vi "Session open.vi"(8 "error in":errorcluster, 11 "measurement configuration":T1={"INTERFACE NAME CAN"="", "IO Mode CAN"=enum."CAN", "FD ISO Mode CAN"=enum."ISO", "Termination CAN"=FALSE, "Baudrate CAN"=0, "FD Baudrate CAN"=0, "INTERFACE NAME LIN"="", "Termination LIN"=FALSE, "CAN interface"="", "LIN interface"="", "Network"="", "DLC INDICATOR"=0, "PAYLOAD INDICATOR"=[0, 0, 0, 0, 0, 0, 0, 0, 0, 0, 0, 0, 0, 0, 0, 0, 0, 0, 0, 0, 0, 0, 0, 0, 0, 0, 0, 0, 0, 0, 0, 0, 0, 0, 0, 0, 0, 0, 0, 0, 0, 0, 0, 0, 0, 0, 0, 0, 0, 0, 0, 0, 0, 0, 0, 0, 0, 0, 0, 0, 0, 0, 0, 0], "IDENTIFIER INDICATOR"=0, "Baudrate LIN"=0} {"Baudrate LIN" format="%x"; "IDENTIFIER INDICATOR" format="%x"; "PAYLOAD INDICATOR" format="%x"; "FD Baudrate CAN" format="%x"; "Baudrate CAN" format="%x"}) -> (0 "error out":errorcluster, 3 "session out":refnum<k21>)   [LabVIEW 2025, in "CAN-LIN Frame Generator.lvclass"]
uses:
  CAN-LIN Frame Generator.lvclass
  Measurement Configuration.ctl
  CAN-LIN Frame Generator UI/Toggle.ctl
  <vilib>/xnet/xnet.llb/XNET Create Session (Frame Output Stream).vi
  CAN-LIN Frame Generator.lvclass/CAN-LIN Frame Generator.ctl
  <resource>/objmgr/xnet.rc
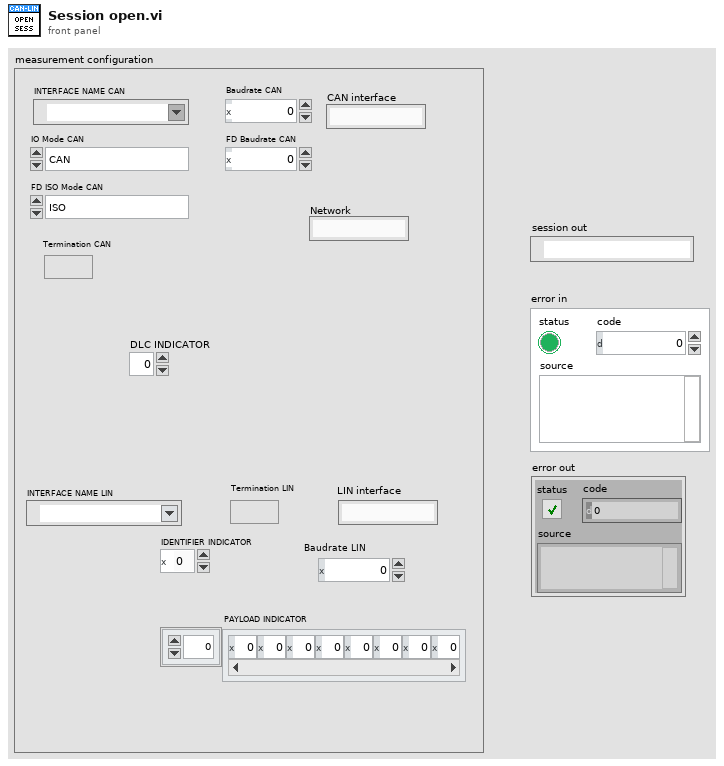
[diagram p1: front panel]
types:
  T1 = typedef "CAN-LIN Frame Generator.lvclass/Measurement Configuration.ctl" = cluster{"INTERFACE NAME CAN":refnum<k21>, "IO Mode CAN":enum32{"CAN", "CAN FD", "CAN FD + BRS"}, "FD ISO Mode CAN":enum32{"ISO", "Legacy ISO", "Non-ISO"}, "Termination CAN":T2, "Baudrate CAN":u32, "FD Baudrate CAN":u32, "INTERFACE NAME LIN":refnum<k21>, "Termination LIN":T2, "CAN interface":string, "LIN interface":string, "Network":string, "DLC INDICATOR":u32, "PAYLOAD INDICATOR":u32[], "IDENTIFIER INDICATOR":u32, "Baudrate LIN":u32}
  T2 = typedef "Toggle.ctl" = bool
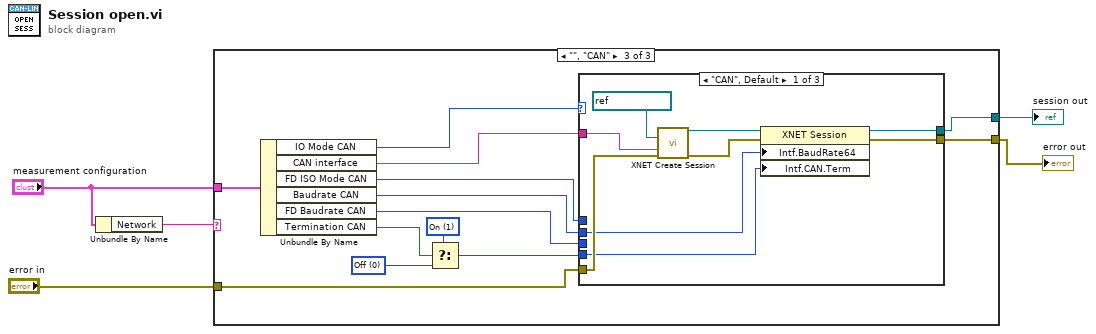
[diagram p0: block diagram]
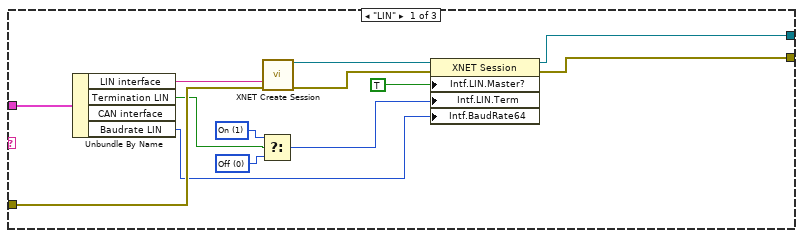
[diagram p2: hidden frame]
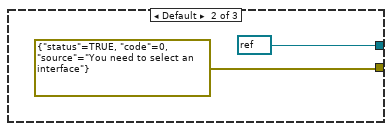
[diagram p3: hidden frame]
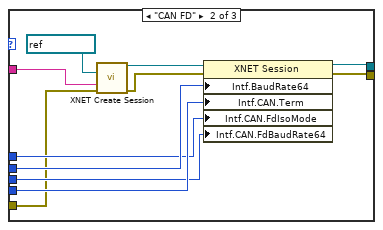
[diagram p4: hidden frame]
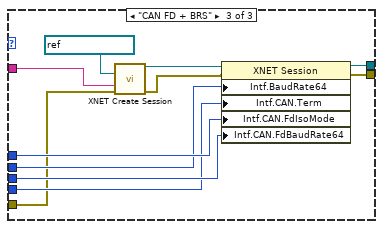
[diagram p5: hidden frame]
diagram:
  n1 = Unbundle By Name("measurement configuration") -> ("Network"=w1:string)
  n2 = case shown="\"\", \"CAN\"" w1 {
    tunnel: "error in" -> [w16 _ w30]
    tunnel: [w8 refnum<k21> refnum ("session out") w23] -> w4
    tunnel: [w7 errorcluster {"status"=TRUE, "code"=0, "source"="You need to select an interface"} ("error out") w22] -> w3
    tunnel: "measurement configuration" -> [w18 _ w21]
    frame "LIN" {
      w11 = u32 0 items=["Off", "On"] ("Interface:LIN:Termination")
      w12 = u32 1 items=["Off", "On"] ("Interface:LIN:Termination")
      n3 = Unbundle By Name(w18) -> ("LIN interface"=w17:string, "Termination LIN"=w13:T2, "Baudrate LIN"=w6:u32)  [unwired: 1 out]
      n4 = Select(t=w12, s=w13, f=w11) -> (s? t:f=w10:u32)
      n5 = call-poly <vilib>:"XNET Create Session.vi"("interface"=w17, "error in (no error)"=w16) -> ("session out"=w15:refnum<k21>, "error out"=w9:errorcluster)  [unwired: 12 in]
      n6 = property class="XNET Session"(reference=w15, error in=w9, "Intf.LIN.Master?"=TRUE ("Interface:LIN:Master?"), "Intf.LIN.Term"=w10, "Intf.BaudRate64"=w6) -> (reference out=w8:refnum<k21>, error out=w7:errorcluster)
    }
    frame Default {
    }
    frame "", "CAN" {
      w28 = u32 0 items=["Off", "On"] ("Interface:CAN:Termination")
      w29 = u32 1 items=["Off", "On"] ("Interface:CAN:Termination")
      n7 = Unbundle By Name(w21) -> ("IO Mode CAN"=w33:enum32{"CAN", "CAN FD", "CAN FD + BRS"}, "CAN interface"=w31:string, "FD ISO Mode CAN"=w25:enum32{"ISO", "Legacy ISO", "Non-ISO"}, "Baudrate CAN"=w26:u32, "FD Baudrate CAN"=w24:u32, "Termination CAN"=w32:T2)
      n8 = Select(t=w29, s=w32, f=w28) -> (s? t:f=w27:u32)
      n9 = case shown="\"CAN\", Default" w33 {
        tunnel: w31 -> [w34 w52 w58]
        tunnel: w30 -> [w42 w46 w57]
        tunnel: w27 -> [w40 w49 w59]
        tunnel: w26 -> [w35 w50 w61]
        tunnel: w25 -> [_ w48 w62]
        tunnel: w24 -> [_ w47 w60]
        tunnel: [w38 w44 w55] -> w22
        tunnel: [w37 w43 w54] -> w23
        frame "CAN", Default {
          n10 = call-poly <vilib>:"XNET Create Session.vi"("cluster (:memory:)"=refnum<k21> ":memory:", "interface"=w34, "error in (no error)"=w42) -> ("session out"=w41:refnum<k21>, "error out"=w39:errorcluster)  [unwired: 11 in]
          n11 = property class="XNET Session"(reference=w41, error in=w39, "Intf.BaudRate64"=w35, "Intf.CAN.Term"=w40) -> (reference out=w37:refnum<k21>, error out=w38:errorcluster)
        }
        frame "CAN FD" {
          n12 = call-poly <vilib>:"XNET Create Session.vi"("cluster (:memory:)"=refnum<k21> ":can_fd:", "interface"=w52, "error in (no error)"=w46) -> ("session out"=w53:refnum<k21>, "error out"=w45:errorcluster)  [unwired: 11 in]
          n13 = property class="XNET Session"(reference=w53, error in=w45, "Intf.BaudRate64"=w50, "Intf.CAN.Term"=w49, "Intf.CAN.FdIsoMode"=w48, "Intf.CAN.FdBaudRate64"=w47) -> (reference out=w43:refnum<k21>, error out=w44:errorcluster)
        }
        frame "CAN FD + BRS" {
          n14 = call-poly <vilib>:"XNET Create Session.vi"("cluster (:memory:)"=refnum<k21> ":can_fd_brs:", "interface"=w58, "error in (no error)"=w57) -> ("session out"=w64:refnum<k21>, "error out"=w56:errorcluster)  [unwired: 11 in]
          n15 = property class="XNET Session"(reference=w64, error in=w56, "Intf.BaudRate64"=w61, "Intf.CAN.Term"=w59, "Intf.CAN.FdIsoMode"=w62, "Intf.CAN.FdBaudRate64"=w60) -> (reference out=w54:refnum<k21>, error out=w55:errorcluster)
        }
      }
    }
  }
  "session out" <- w4
  "error out" <- w3
